vi "UI Event Holder.vi"() -> ()   [LabVIEW 2015]
uses:
  <vilib>/Utility/miscctls.llb/LVPoint32TypeDef.ctl
panel:
  out "Coords":T1
  in  "Time Ceck":bool
  out "current time":timestamp
  out "Iteration":i32
  in  "Stop":bool
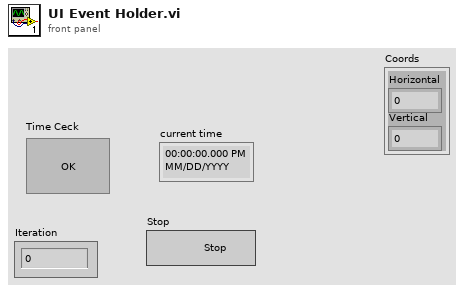
[diagram p1: front panel]
types:
  T1 = typedef "LVPoint32TypeDef.ctl" = cluster{"Horizontal":i32, "Vertical":i32}
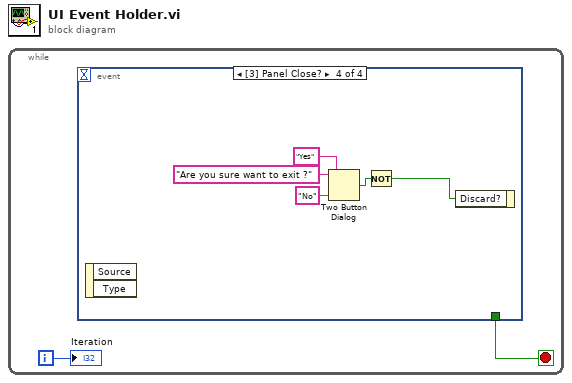
[diagram p0: block diagram]
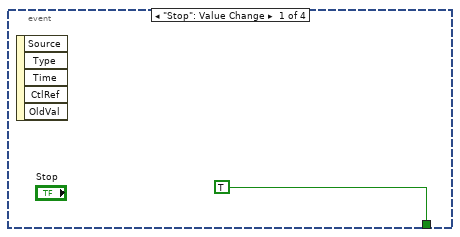
[diagram p2: hidden frame]
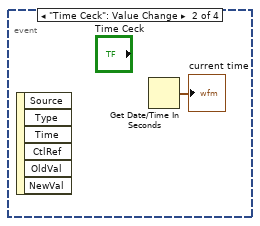
[diagram p3: hidden frame]
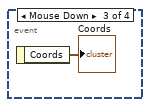
[diagram p4: hidden frame]
diagram:
  n1 = while {
    i -> [w2]
    stop <- w1 stop-if-true
    n2 = event shown="[3] Panel Close?" {
      selector: _ -> [_ _ _ _]
      dyn-events: _ -> [_ _ _ _]
      timeout: _ -> [_ _ _ _]
      tunnel: [TRUE _ _ _] -> w1
      event "Stop": Value Change {
        n3 = event-data() -> ()  [unwired: 1 in, 5 out]
      }
      event "Time Ceck": Value Change {
        n4 = event-data() -> ()  [unwired: 1 in, 6 out]
        n5 = Get Date/Time In Seconds() -> (seconds since 1Jan1904=→"current time":timestamp)
      }
      event Mouse Down {
        n6 = event-data() -> ("Coords"=→"Coords":T1)  [unwired: 1 in]
      }
      event Panel Close? {
        n7 = event-data() -> ()  [unwired: 1 in, 2 out]
        n8 = Two Button Dialog(message="Are you sure want to exit ?", 1:"No" ("F button name (\"Cancel\")"), 2:"Yes" ("T button name (\"OK\")")) -> (T button?=w9:bool)
        n9 = Not(x=w9) -> (.not. x?=w10:bool)
        n10 = event-data("Discard?"=w10) -> ()  [unwired: 1 in, 1 out]
      }
    }
    "Iteration" <- w2
  }
